vi "GOOP4_Sub_Implement.vi"(11 "ClassThatImplements":refnum<class "GOOP4_Sub.lvclass">) -> (3 "InterfaceHelpClass":refnum<class "GOOP4_Sub_AAAa.lvclass">)   [LabVIEW 2019, in "GOOP4_Sub_AAAa.lvclass"]
doc: "Implemnts an Interface"
uses:
  GOOP4_Sub_AAAa.lvclass
  GOOP4_Sub_class/GOOP4_Sub.lvclass
  GOOP4_Sub_AAAa.lvclass/GOOP4_Sub_AAAa.ctl
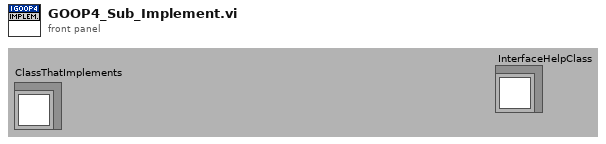
[diagram p1: front panel]
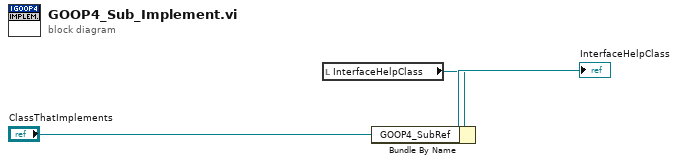
[diagram p0: block diagram]
diagram:
  n1 = local read "InterfaceHelpClass"() -> (w1:refnum<class "GOOP4_Sub_AAAa.lvclass">)
  n2 = Bundle By Name(cluster=w1, "GOOP4_SubRef"="ClassThatImplements") -> (→"InterfaceHelpClass":refnum<class "GOOP4_Sub_AAAa.lvclass">)
